vi "ParseInvalidCofigurationMessage.vi"(8 "error in (no error)":errorcluster, 11 "process error message":variant) -> (0 "error out":errorcluster, 2 "description":string)   [LabVIEW 2017, in "Qbus.lvclass"]
uses:
  <vilib>/addons/Qbus/Qbus.lvclass
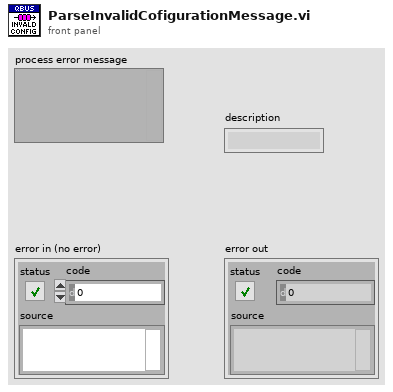
[diagram p1: front panel]
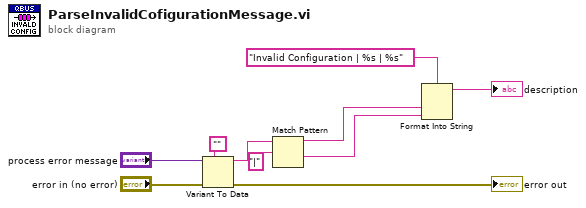
[diagram p0: block diagram]
diagram:
  n1 = Variant To Data(error in="error in (no error)", type="", Variant="process error message") -> (data=w4:string, error out=→"error out":errorcluster)
  n2 = Match Pattern(string=w4, regular expression="|" ("string")) -> (before substring=w3:string, after substring=w2:string)  [unwired: 1 in, 2 out]
  n3 = Format Into String(format string="Invalid Configuration | %s | %s", w3, w2) -> (resulting string=→"description":string)  [unwired: 2 in, 1 out]
